vi "countrate.vi"() -> ()   [LabVIEW 2015]
doc: "This program functinons as a count-rate meter that allows the user to control the total count time, count interval, and the output file name. The program displays the counts vs. time at the end of the program run."
uses:
  <vilib>/Platform/TimedLoop/XDataNode/timing_clust.ctl
  <vilib>/Platform/TimedLoop/XDataNode/nitl_modes.ctl
  <vilib>/Platform/TimedLoop/XDataNode/wakeup.ctl
  <vilib>/Utility/file.llb/Write Delimited Spreadsheet (I64).vi
  <vilib>/platform/TimedLoop/XDataNode/XDataNode.xnode
  <vilib>/Platform/TimedLoop/XDataNode/XDNodeRunTimeDep.lvlib
panel:
  out "status":cluster{"Time Elapsed (sec)":dbl, "Counts":dbl} caption="COUNTING STATUS"
  out "XY Graph":cluster{i32[], i32[]}(graph)
  in  "File Path Control":path
  in  "controls":cluster{"Total Time":i32, "Cnt Interval":i32} caption="USER CONTROLS"
  in  "Stop Button":bool
  out "counts per interval":dbl(knob) scale=0.0..100.0
  # "Demo count rate VI for Physics 434"
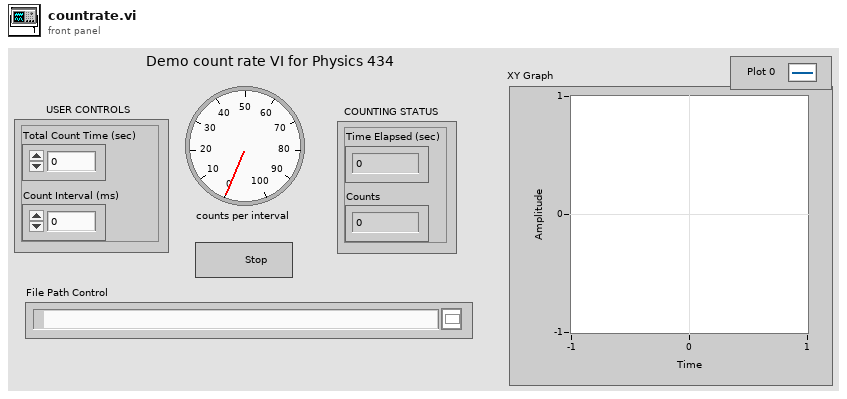
[diagram p1: front panel]
types:
  T1 = typedef "XDNodeRunTimeDep.lvlib/timing_clust.ctl" = cluster{"Expected End [f-1]":u64, "Actual End [f-1]":u64, "Finished Late? [f-1]":bool, "Expected End [i-1]":u64, "Actual End [i-1]":u64, "Finished Late? [i-1]":bool, "Expected Start [i]":u64, "Actual Start [i]":u64, "Expected Start [f]":u64, "Actual Start [f]":u64, "Source Name":string, "Structure Name":string, "Period":i64, "Deadline":i64, "Offset":i64, "Start":i64, "Priority":i32, "Timeout":i32, "Mode":T2, "Wakeup Reason":T3, "Error":errorcluster, "Source Type":string, "Secondary Source Type":string, "Global End Time":u64, "Global Start Time":u64, "Frame Duration":u64, "Iteration Duration":u64, "Assigned CPU":i32, "I/O Scan Engine Mode":u32}
  T2 = typedef "XDNodeRunTimeDep.lvlib/nitl_modes.ctl" = enum32{"No Change", "Process missed periods, maintain original phase", "Discard missed periods, maintain original phase", "Process missed periods, ignore original phase", "Discard missed periods, ignore original phase"}
  T3 = typedef "XDNodeRunTimeDep.lvlib/wakeup.ctl" = enum32{"Normal", "Aborted", "Asynchronous wakeup", "Timing source error", "Timed loop error", "Timeout"}
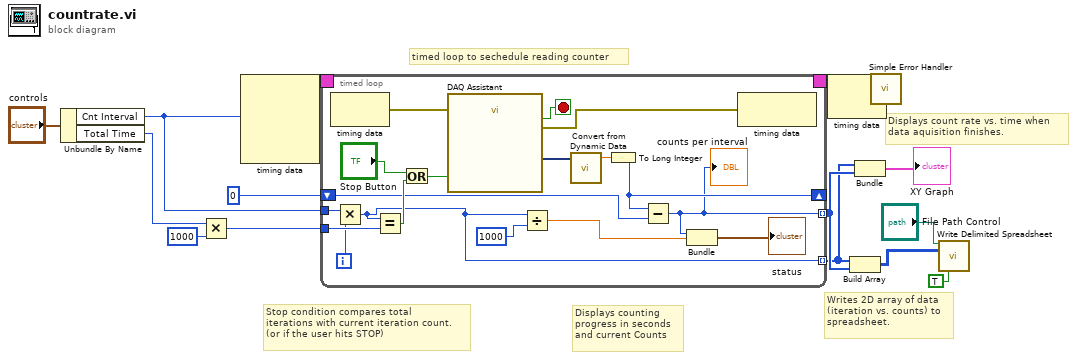
[diagram p0: block diagram]
diagram:
  # "Displays counting \nprogress in seconds \nand current Counts"
  # "Writes 2D array of data \n(iteration vs. counts) to \nspreadsheet."
  # "Displays count rate vs. time when \ndata aquisition finishes."
  # "Stop condition compares total \niterations with current iteration count. \n(or if the user hits STOP)"
  # "timed loop to sechedule reading counter"
  n1 = Unbundle By Name("controls") -> ("Cnt Interval"=w8:i32, "Total Time"=w10:i32)
  n2 = Multiply(x=w10, y=i64 1000) -> (x*y=w7:i64)
  n3 = node-c288(w8) -> (w15:T1)  [unwired: 3 in]
  n4 = timed-loop {
    timing: w15 -> [_]
    timing-out: [_] -> w14
    shift-right: [w31] -> _
    shift-left: 0 -> [w20]
    tunnel: w8 -> [w25]
    tunnel: w7 -> [w24]
    tunnel: [w17] -> w2 mode=indexing
    tunnel: [w19] -> w1 mode=indexing
    i -> [w22]
    stop <- w32 stop-if-true
    n5 = node-c288() -> (w28:errorcluster)  [unwired: 1 in]
    n6 = Multiply(x=w25, y=w22) -> (x*y=w19:i32)
    n7 = Equal?(x=w19, y=w24) -> (x = y?=w23:bool)
    n8 = Or(x="Stop Button", y=w23) -> (x .or. y?=w27:bool)
    n9 = call "DAQ Assistant"("error in"=w28, "stop (F)"=w27) -> ("data"=w33:dynamicdata, "stopped"=w32:bool, "error out"=w29:errorcluster)  [unwired: 14 in, 1 out]
    n10 = Divide(x=w19, y=1000) -> (x/y=w16:dbl)
    n11 = call "Convert from Dynamic Data"("Dynamic Data Type"=w33) -> ("Scalar"=w30:dbl)  [unwired: 3 in]
    n12 = To Long Integer(number=w30) -> (32bit integer=w31:i32)
    n13 = Subtract(x=w31, y=w20) -> (x-y=w17:i32)
    "counts per interval" <- w17
    n14 = Bundle(w17, w16) -> (→"status":cluster{i32, dbl})  [unwired: 1 in]
    n15 = node-c288(w29) -> ()  [unwired: 1 out]
  }
  n16 = node-c288(w14) -> (w12:errorcluster)
  n17 = Build Array(w1, w2) -> (w3:i32[][])
  n18 = Bundle(w1, w2) -> (→"XY Graph":cluster{i32[], i32[]})  [unwired: 1 in]
  n19 = call <vilib>:"Simple Error Handler.vi"("error in (no error)"=w12) -> ()  [unwired: 4 in, 5 out]
  n20 = call-poly <vilib>:"Write Delimited Spreadsheet.vi"("file path (dialog if empty)"="File Path Control", "2D data"=w3, "transpose? (F)"=TRUE) -> ()  [unwired: 11 in, 2 out]
